vi "CD Init_Prepare Inline Data_Fill Frame Descriptors from BC configuration.vi"(8 "error in (no error)":errorcluster, 11 "RT Channel In":T1 {"RTs"."Mode Codes"."Words Item Refs" format="%.0x"; "RTs"."Mode Codes"."Words Block Data Refs"."Data Reference" format="%.0x"; "RTs"."Mode Codes"."Timestamp Channel Data Reference" format="%.0x"; "RTs"."subAddresses"."Words Item Refs" format="%.0x"; "RTs"."subAddresses"."Words Block Data Refs"."Data Reference" format="%.0x"; "RTs"."subAddresses"."Timestamp Channel Data Reference" format="%.0x"; "RTs"."Status Channel Data Reference" format="%.0x"; "RTs"."Command Channels Refs" format="%.0x"; "BC"."Acyclic Frames Trigger Channels Refs" format="%.0x"; "BC"."Command Channels Refs" format="%.0x"; "BC"."messages"."Timestamp Channel Data Reference" format="%.0x"; "BC"."messages"."Status Channel Data Refs" format="%.0x"; "BC"."messages"."Words Item Refs" format="%.0x"; "BC"."messages"."Words Block Data Refs"."Data Reference" format="%.0x"}) -> (0 "error out":errorcluster, 2 "RTs":T10[](array[typedef]) {"Mode Codes"."Words Item Refs" format="%.0x"; "Mode Codes"."Words Block Data Refs"."Data Reference" format="%.0x"; "Mode Codes"."Timestamp Channel Data Reference" format="%.0x"; "subAddresses"."Words Item Refs" format="%.0x"; "subAddresses"."Words Block Data Refs"."Data Reference" format="%.0x"; "subAddresses"."Timestamp Channel Data Reference" format="%.0x"; "Status Channel Data Reference" format="%.0x"; "Command Channels Refs" format="%.0x"}, 3 "Frames Descriptors Out":T15[](array[typedef]) {"RT"."Status Channel Ref" format="%.0x"; "RT"."Words Block Data Refs"."Data Reference" format="%.0x"; "RT"."Timestamp Channel Data Reference" format="%.0x"; "BC"."Status Channel Refs" format="%.0x"; "BC"."Words Block Data Refs"."Data Reference" format="%.0x"; "BC"."Timestamp Channel Data Reference" format="%.0x"})   [LabVIEW 2017, in "Ballard MIL-1553 Engine.lvlib"]
uses:
  Ballard MIL-1553 Engine.lvlib
  Controls/RT Inline Frame Descriptor.ctl
  Controls/RT Inline Frame Descriptor_BC.ctl
  <vilib>/NI Veristand/Custom Device API/Data Reference.ctl
  <vilib>/NI Veristand/Custom Device API/Block Data Reference.ctl
  <vilib>/NI Veristand/Custom Device API/Custom Device Item Ref.ctl
  Controls/RT Inline Frame Descriptor_RT.ctl
  Shared/Controls and Global/RT CWD2.ctl
  Shared/Controls and Global/RT CWD1.ctl
  Shared/Controls and Global/RT messageType.ctl
  Shared/Controls and Global/RT Remote Terminal.ctl
  Shared/Controls and Global/RT Remote Terminal_rtMode.ctl
  Shared/Controls and Global/RT Remote Terminal_RT subAddress.ctl
  Shared/Controls and Global/RT Remote Terminal_RT direction.ctl
  Shared/Controls and Global/RT Remote Terminal_RT Mode Code.ctl
  Shared/Controls and Global/RT Channel.ctl
  Shared/Controls and Global/RT BC.ctl
  Shared/Controls and Global/RT Message.ctl
  Shared/Ballard 1553 Shared.lvlib
  <vilib>/NI VeriStand/Custom Device API/Custom Device API.lvlib
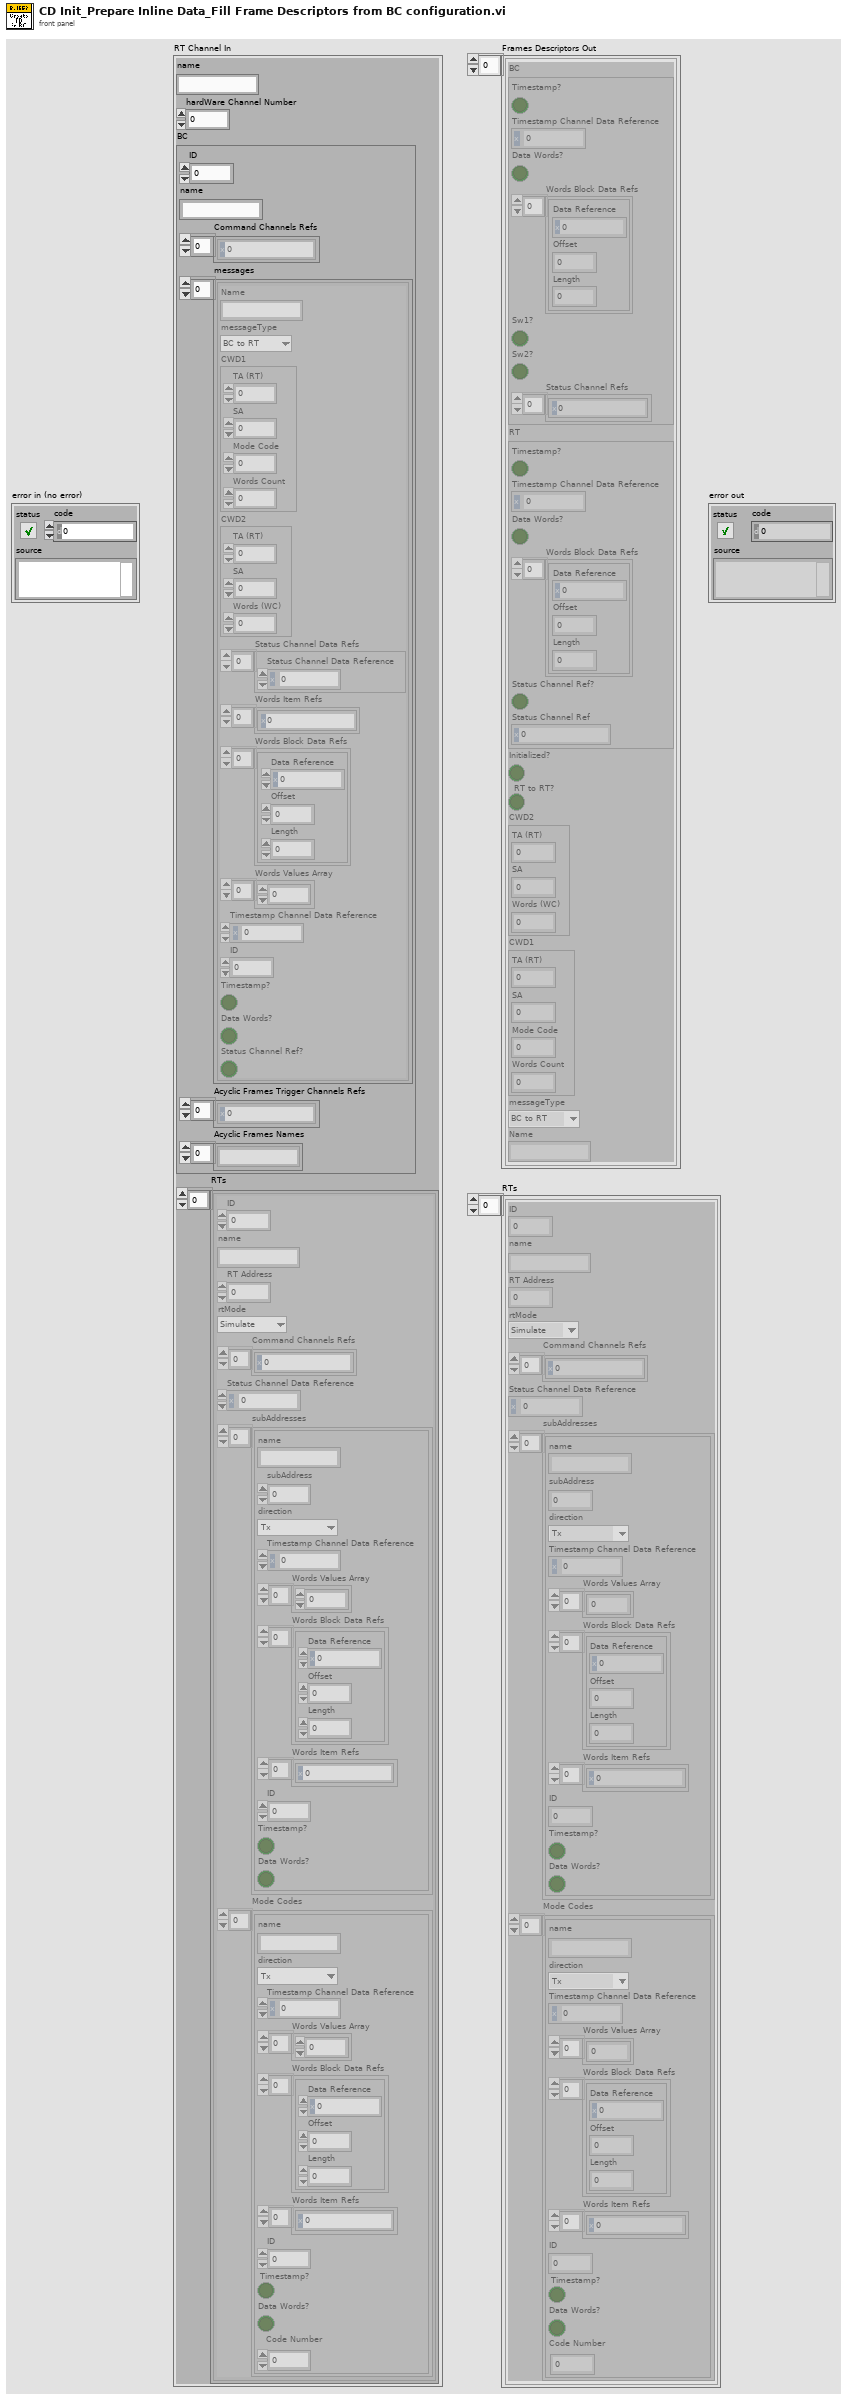
[diagram p1: front panel]
types:
  T1 = typedef "Ballard 1553 Shared.lvlib/RT Channel.ctl" = cluster{"name":string, "hardWare Channel Number":u16, "BC":T2, "RTs":T10[]}
  T2 = typedef "Ballard 1553 Shared.lvlib/RT BC.ctl" = cluster{"ID":i32, "name":string, "Command Channels Refs":T3[], "messages":T4[], "Acyclic Frames Trigger Channels Refs":T3[], "Acyclic Frames Names":string[]}
  T3 = typedef "Custom Device API.lvlib/Custom Device Item Ref.ctl" = u64
  T4 = typedef "Ballard 1553 Shared.lvlib/RT Message.ctl" = cluster{"Name":string, "messageType":T5, "CWD1":T6, "CWD2":T7, "Status Channel Data Refs":T8[], "Words Item Refs":T3[], "Words Block Data Refs":T9[], "Words Values Array":u16[], "Timestamp Channel Data Reference":T8, "ID":i32, "Timestamp?":bool, "Data Words?":bool, "Status Channel Ref?":bool}
  T5 = typedef "Ballard 1553 Shared.lvlib/RT messageType.ctl" = enum16{"BC to RT", "RT to BC", "RT to RT", "MC (Rx)", "MC (Tx)"}
  T6 = typedef "Ballard 1553 Shared.lvlib/RT CWD1.ctl" = cluster{"TA (RT)":i8, "SA":i8, "Mode Code":i8, "Words Count":i8}
  T7 = typedef "Ballard 1553 Shared.lvlib/RT CWD2.ctl" = cluster{"TA (RT)":i8, "SA":i8, "Words (WC)":i8}
  T8 = typedef "Custom Device API.lvlib/Data Reference.ctl" = i32
  T9 = typedef "Custom Device API.lvlib/Block Data Reference.ctl" = cluster{"Data Reference":T8, "Offset":u64, "Length":u64}
  T10 = typedef "Ballard 1553 Shared.lvlib/RT Remote Terminal.ctl" = cluster{"ID":i32, "name":string, "RT Address":i32, "rtMode":T11, "Command Channels Refs":T3[], "Status Channel Data Reference":T8, "subAddresses":T12[], "Mode Codes":T14[]}
  T11 = typedef "Ballard 1553 Shared.lvlib/RT Remote Terminal_rtMode.ctl" = enum16{"Simulate", "Monitor", "Disable"}
  T12 = typedef "Ballard 1553 Shared.lvlib/RT Remote Terminal_RT subAddress.ctl" = cluster{"name":string, "subAddress":i8, "direction":T13, "Timestamp Channel Data Reference":T8, "Words Values Array":u16[], "Words Block Data Refs":T9[], "Words Item Refs":T3[], "ID":i32, "Timestamp?":bool, "Data Words?":bool}
  T13 = typedef "Ballard 1553 Shared.lvlib/RT Remote Terminal_RT direction.ctl" = enum16{"Tx", "Rx"}
  T14 = typedef "Ballard 1553 Shared.lvlib/RT Remote Terminal_RT Mode Code.ctl" = cluster{"name":string, "direction":T13, "Timestamp Channel Data Reference":T8, "Words Values Array":u16[], "Words Block Data Refs":T9[], "Words Item Refs":T3[], "ID":i32, "Timestamp?":bool, "Data Words?":bool, "Code Number":i32}
  T15 = typedef "Ballard MIL-1553 Engine.lvlib/RT Inline Frame Descriptor.ctl" = cluster{"BC":T16, "RT":T17, "Initialized?":bool, "RT to RT?":bool, "CWD2":T7, "CWD1":T6, "messageType":T5, "Name":string}
  T16 = typedef "Ballard MIL-1553 Engine.lvlib/RT Inline Frame Descriptor_BC.ctl" = cluster{"Timestamp?":bool, "Timestamp Channel Data Reference":T8, "Data Words?":bool, "Words Block Data Refs":T9[], "Sw1?":bool, "Sw2?":bool, "Status Channel Refs":T3[]}
  T17 = typedef "Ballard MIL-1553 Engine.lvlib/RT Inline Frame Descriptor_RT.ctl" = cluster{"Timestamp?":bool, "Timestamp Channel Data Reference":T8, "Data Words?":bool, "Words Block Data Refs":T9[], "Status Channel Ref?":bool, "Status Channel Ref":T3}
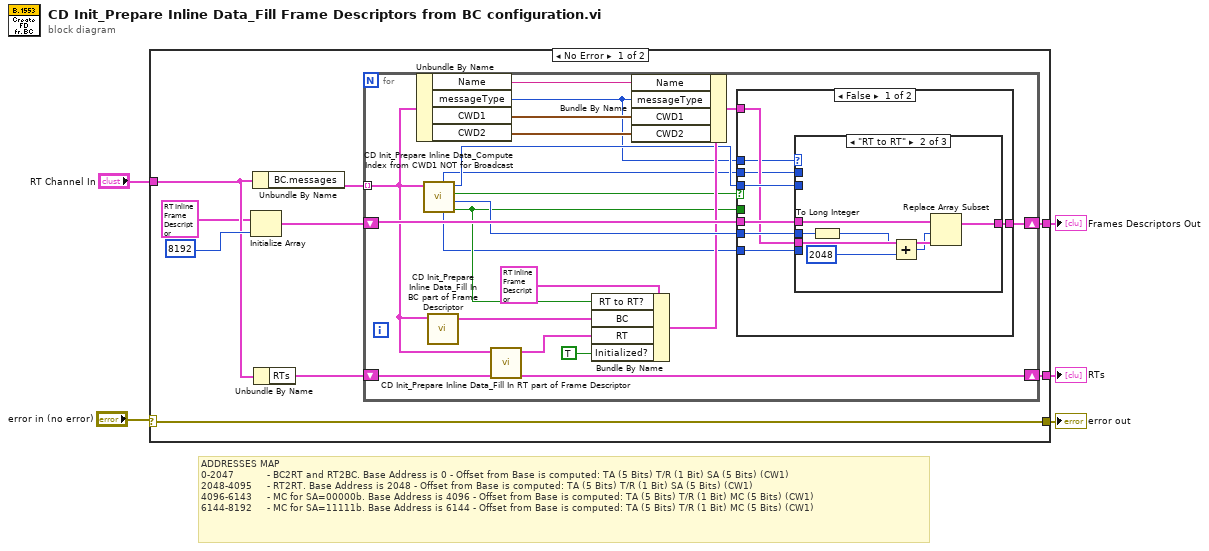
[diagram p0: block diagram]
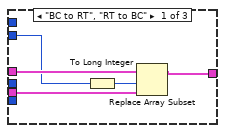
[diagram p2: hidden frame]
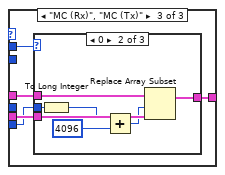
[diagram p3: hidden frame]
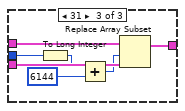
[diagram p5: hidden frame]
diagram:
  # "ADDRESSES MAP \n0-2047           - BC2RT and RT2BC. Base Address is 0 - Offset from Base is computed: TA (5 Bits) T/R (1 Bit) SA (5 Bits) (CW1)\n2048-4095     - RT2RT. Base Address is 2048 - Offset from Base is computed: TA (5 Bits) T/R (1 Bit) SA (5 Bits) (CW1)\n4096-6143     - MC for SA=00000b. Base Address is 4096 - Offset from Base is computed: TA (5 Bits) T/R (1 Bit) MC (5 Bits) (CW1)\n6144-8192     - MC for SA=11111b. Base Address is 6144 - Offset from Base is computed: TA (5 Bits) T/R (1 Bit) MC (5 Bits) (CW1)"
  n1 = case shown="No Error" "error in (no error)" {
    selector: "error in (no error)" -> [w6 w77]
    tunnel: [w13 _] -> w5
    tunnel: [w12 _] -> w4
    tunnel: "RT Channel In" -> [w10 _]
    tunnel: [w6 w77] -> w1
    frame No Error {
      n2 = Initialize Array(T15 {"BC"={"Timestamp?"=FALSE, "Timestamp Channel Data Reference"=0, "Data Words?"=FALSE, "Words Block Data Refs"=[], "Sw1?"=FALSE, "Sw2?"=FALSE, "Status Channel Refs"=[]}, "RT"={"Timestamp?"=FALSE, "Timestamp Channel Data Reference"=0, "Data Words?"=FALSE, "Words Block Data Refs"=[], "Status Channel Ref?"=FALSE, "Status Channel Ref"=0}, "Initialized?"=FALSE, "RT to RT?"=FALSE, "CWD2"={"TA (RT)"=0, "SA"=0, "Words (WC)"=0}, "CWD1"={"TA (RT)"=0, "SA"=0, "Mode Code"=0, "Words Count"=0}, "messageType"=enum."BC to RT", "Name"=""} ("Frame Descriptor"), 8192 ("dimension size")) -> (w8:T15[])
      n3 = Unbundle By Name(w10) -> ("BC.messages"=w9:T4[])
      n4 = Unbundle By Name(w10) -> ("RTs"=w11:T10[])
      n5 = for {
        shift-right: [w34] -> w13
        shift-left: w8 -> [w35]
        tunnel: w9 -> [w22] mode=indexing
        shift-right: [w19] -> w12
        shift-left: w11 -> [w30]
        n6 = Unbundle By Name(w22) -> ("Name"=w26:string, "messageType"=w17:T5, "CWD1"=w25:T6, "CWD2"=w24:T7)
        n7 = call "CD Init_Prepare Inline Data_Compute Index from CWD1 NOT for Broadcast.vi"("message"=w22) -> ("RT to RT?"=w20:bool, "Index 1"=w28:u32, "Broadcast?"=w18:bool, "Index 0"=w23:u16, "Index 2"=w16:u16, "CWD1.SA"=w15:i8)  [unwired: 5 in]
        n8 = call "CD Init_Prepare Inline Data_Fill In BC part of Frame Descriptor.vi"("message"=w22) -> ("BC Frame Descriptor"=w32:T16)  [unwired: 10 in]
        n9 = call "CD Init_Prepare Inline Data_Fill In RT part of Frame Descriptor.vi"("RTs In"=w30, "message"=w22) -> ("RTs Out"=w19:T10[], "RT Frame Descriptor"=w31:T17)  [unwired: 8 in]
        n10 = Bundle By Name(cluster=T15 {"BC"={"Timestamp?"=FALSE, "Timestamp Channel Data Reference"=0, "Data Words?"=FALSE, "Words Block Data Refs"=[], "Sw1?"=FALSE, "Sw2?"=FALSE, "Status Channel Refs"=[]}, "RT"={"Timestamp?"=FALSE, "Timestamp Channel Data Reference"=0, "Data Words?"=FALSE, "Words Block Data Refs"=[], "Status Channel Ref?"=FALSE, "Status Channel Ref"=0}, "Initialized?"=FALSE, "RT to RT?"=FALSE, "CWD2"={"TA (RT)"=0, "SA"=0, "Words (WC)"=0}, "CWD1"={"TA (RT)"=0, "SA"=0, "Mode Code"=0, "Words Count"=0}, "messageType"=enum."BC to RT", "Name"=""} ("Frame Descriptor"), "RT to RT?"=w20, "BC"=w32, "RT"=w31, "Initialized?"=TRUE) -> (w27:T15)
        n11 = Bundle By Name(cluster=w27, "Name"=w26, "messageType"=w17, "CWD1"=w25, "CWD2"=w24) -> (w21:T15)
        n12 = case shown="False" w18 {
          tunnel: w35 -> [w43 w76]
          tunnel: [w42 w76] -> w34
          tunnel: w28 -> [w41 _]
          tunnel: w23 -> [w40 _]
          tunnel: w21 -> [w39 _]
          tunnel: w20 -> [_ _]
          tunnel: w17 -> [w38 _]
          tunnel: w16 -> [w36 _]
          tunnel: w15 -> [w37 _]
          frame False {
            n13 = case shown="\"RT to RT\"" w38 {
              tunnel: w43 -> [w48 w55 w60]
              tunnel: [w47 w54 w59] -> w42
              tunnel: w41 -> [_ w50 _]
              tunnel: w39 -> [w45 w53 w58]
              tunnel: w40 -> [w44 _ _]
              tunnel: w37 -> [_ _ w57]
              tunnel: w36 -> [_ _ w56]
              frame "BC to RT", "RT to BC" {
                n14 = To Long Integer(number=w44) -> (32bit integer=w46:i32)
                n15 = Replace Array Subset(array=w48, new element=w45, index=w46) -> (w47:T15[])
              }
              frame "RT to RT" {
                n16 = To Long Integer(number=w50) -> (32bit integer=w52:i32)
                n17 = Add(x=w52, y=2048) -> (x+y=w51:i32)
                n18 = Replace Array Subset(array=w55, new element=w53, index=w51) -> (w54:T15[])
              }
              frame "MC (Rx)", "MC (Tx)" {
                n19 = case shown="0" w57 {
                  tunnel: w60 -> [w61 w68 w75]
                  tunnel: [w61 w67 w74] -> w59
                  tunnel: w58 -> [_ w66 w73]
                  tunnel: w56 -> [_ w63 w70]
                  frame 1, Default {
                  }
                  frame 0 {
                    n20 = To Long Integer(number=w63) -> (32bit integer=w65:i32)
                    n21 = Add(x=w65, y=4096) -> (x+y=w64:i32)
                    n22 = Replace Array Subset(array=w68, new element=w66, index=w64) -> (w67:T15[])
                  }
                  frame 31 {
                    n23 = To Long Integer(number=w70) -> (32bit integer=w72:i32)
                    n24 = Add(x=w72, y=6144) -> (x+y=w71:i32)
                    n25 = Replace Array Subset(array=w75, new element=w73, index=w71) -> (w74:T15[])
                  }
                }
              }
            }
          }
          frame True {
          }
        }
      }
    }
    frame Error {
    }
  }
  "Frames Descriptors Out" <- w5
  "RTs" <- w4
  "error out" <- w1
